vi "RSMA Receiver - 2 Channels - Kopie.vi"() -> ()   [LabVIEW 2022 SP3]
panel:
  out "W2":string
  out "W1":string
  out "Constellation Map":cluster{"Constellation":cdb[]}[](graph)
  in  "Tab Control":enum32{"USRP Parameters", "Rx Info", "BER"}(tab)
  in  "USRP ControledParameters":T1={"Active Antenna"="RX2", "Gain (dB)"=0.0, "Carrier Frequency"=2400000000.0, "IQ Rate"=2000000.0, "Active channels"="0,1"} {"IQ Rate" format="%#_6p"; "Carrier Frequency" format="%#_6p"; "Gain (dB)" format="%#_6f"}
  in  "Device selection":refnum<k15>="RIO0"
  in  "Trigger level":dbl=0.01 format="%f"
  out "SIG valid? - CH1":bool
  out "SIG valid? - CH0":bool
  out "Frequency offset - CH1":dbl
  out "Frequency offset - CH0":dbl
  out "Coerced Parameters":T2={"IQ Rate"=100000.0, "Carrier  Freq."=100000.0, "Gain"=0.0} {"Gain" format="%#_6f"; "Carrier  Freq." format="%#_6p"; "IQ Rate" format="%#_6p"}
  out "Error out":errorcluster
  in  "Record BER":bool
  out "No. Bits - CH0":dbl format="%#_6f"
  out "No. Bits - CH1":dbl
  in  "error in (no error)":errorcluster
  # "RSMA Receiver"
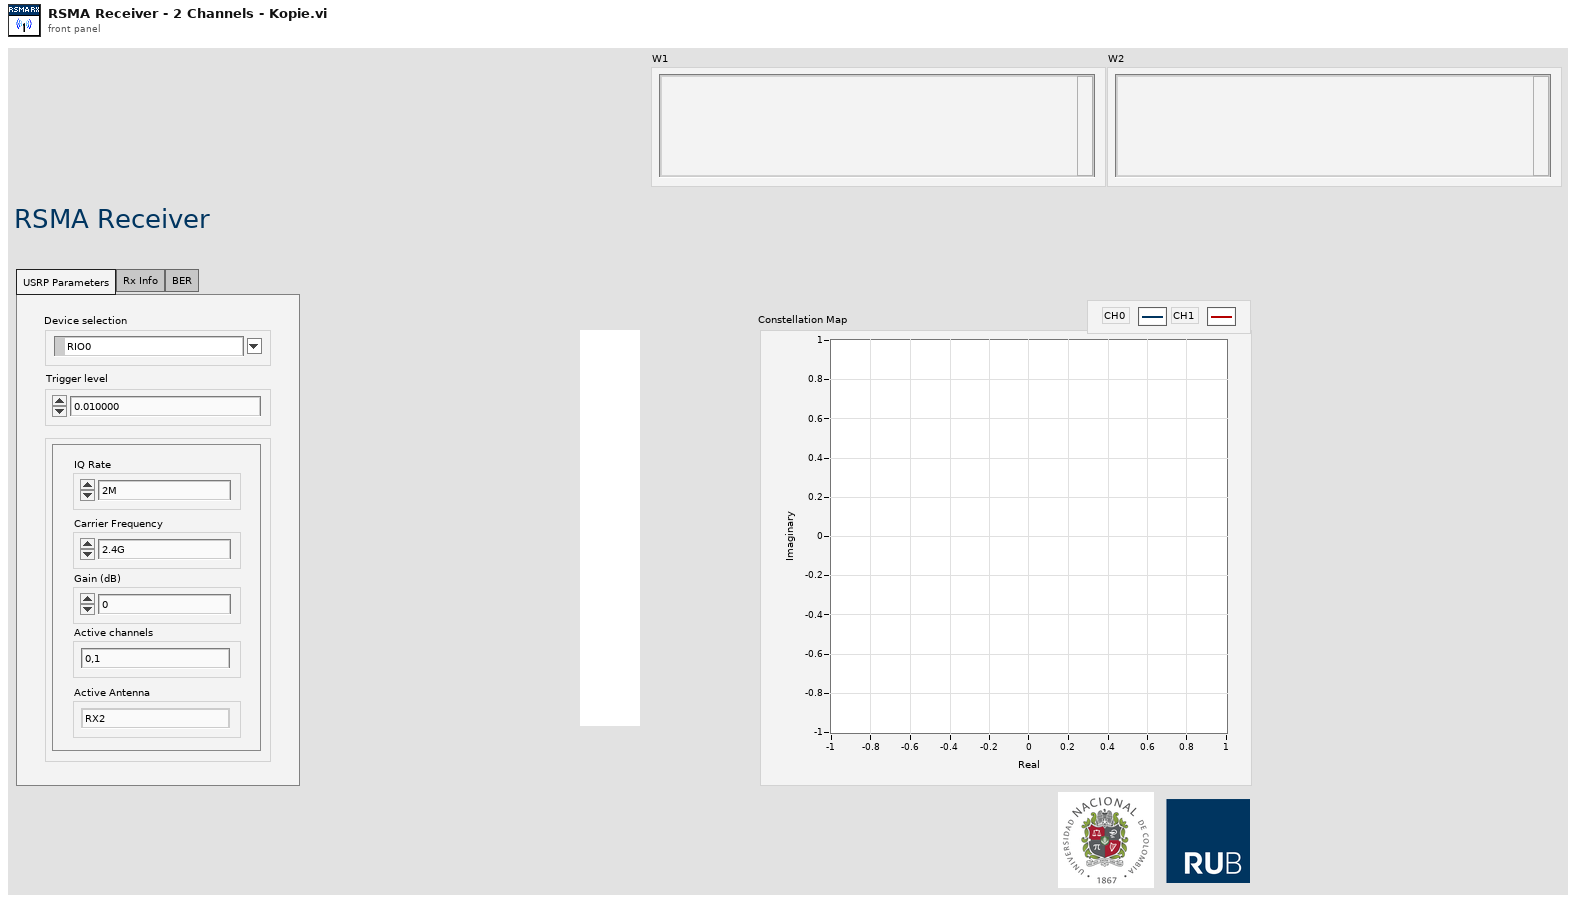
[diagram p1: front panel]
types:
  T1 = cluster{"Active Antenna":string, "Gain (dB)":dbl, "Carrier Frequency":dbl, "IQ Rate":dbl, "Active channels":string}
  T2 = cluster{"IQ Rate":dbl, "Carrier  Freq.":dbl, "Gain":dbl}
  T3 = cluster{"coerced IQ rate":dbl, "coerced carrier frequency":dbl, "coerced gain":dbl}
  T4 = cluster{"Modulation type":enum16{"QPSK(4QAM)", "64QAM", "16QAM", "BPSK"}, "BCC rate (k/n)":enum16{"1/2", "2/3", "3/4"}}
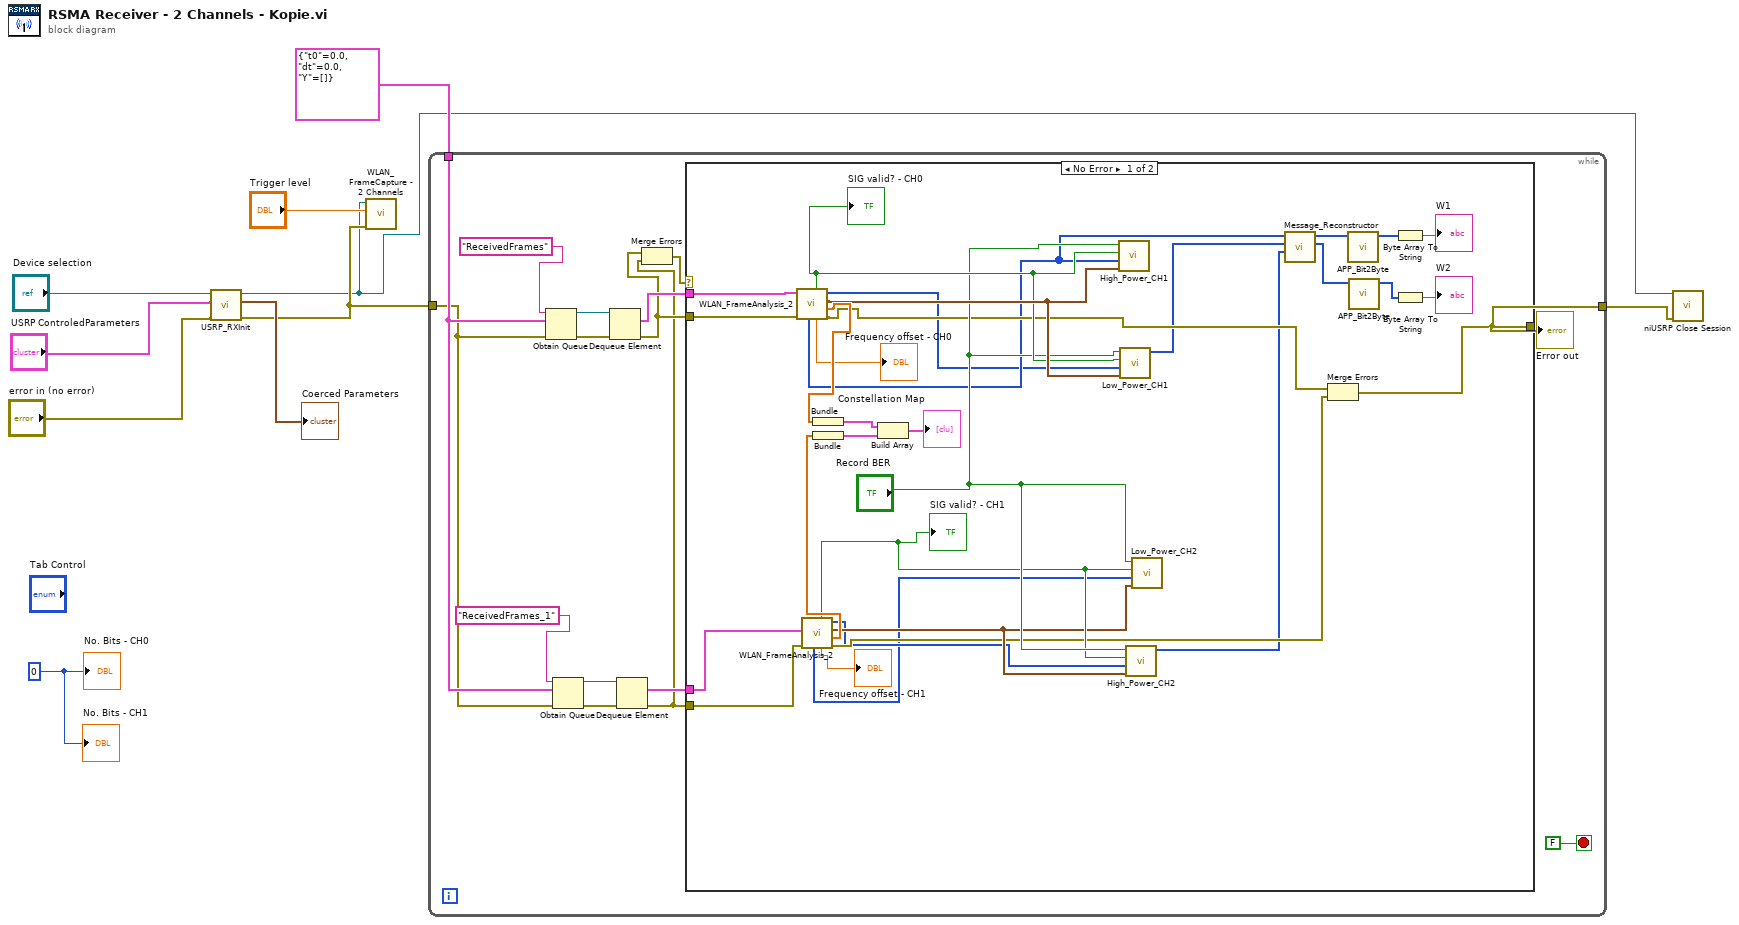
[diagram p0: block diagram]
diagram:
  w1 = 0
  n1 = call "USRP_RXInit.vi"("device names"="Device selection", "USRP ControledParameters"="USRP ControledParameters", "error in (no error)"="error in (no error)") -> ("session handle out"=w4:refnum<k15>, "USRP CoercedParamters"=→"Coerced Parameters":T3, "error out"=w8:errorcluster)  [unwired: 5 in]
  n2 = call "WLAN_FrameCapture - 2 Channels.vi"("error in (no error)"=w8, "Trigger level"="Trigger level", "session handle"=w4) -> ()  [unwired: 8 in]
  n3 = while {
    tunnel: w8 -> [w16]
    tunnel: cluster{"t0":dbl, "dt":dbl, "Y":cdb[]} {"t0"=0.0, "dt"=0.0, "Y"=[]} ("data") -> [w17]
    tunnel: [w21] -> w5
    stop <- FALSE stop-if-true
    n4 = Obtain Queue(name (unnamed)="ReceivedFrames", element data type=w17, error in (no error)=w16) -> (queue out=w25:refnum<queue>, error out=w23:errorcluster)  [unwired: 2 in, 1 out]
    n5 = Obtain Queue(name (unnamed)="ReceivedFrames_1", element data type=w17, error in (no error)=w16) -> (queue out=w20:refnum<queue>, error out=w19:errorcluster)  [unwired: 2 in, 1 out]
    n6 = Dequeue Element(queue=w25, error in (no error)=w23) -> (element=w24:cluster{"t0":dbl, "dt":dbl, "Y":cdb[]}, error out=w13:errorcluster)  [unwired: 1 in, 2 out]
    n7 = Dequeue Element(queue=w20, error in (no error)=w19) -> (element=w15:cluster{"t0":dbl, "dt":dbl, "Y":cdb[]}, error out=w12:errorcluster)  [unwired: 1 in, 2 out]
    n8 = Merge Errors(w13, w12) -> (w11:errorcluster)
    n9 = case shown="No Error" w11 {
      selector: w11 -> [_ w57]
      tunnel: w24 -> [w53 _]
      tunnel: [w38 w57] -> w21
      tunnel: w12 -> [w46 _]
      tunnel: w15 -> [w47 _]
      tunnel: w13 -> [w50 _]
      frame No Error {
        n10 = call "WLAN_FrameAnalysis_2.vi"("error in (no error)"=w50, "input cluster"=w53) -> ("error out"=w39:errorcluster, "Constellation"=w52:cdb[], "Modulation parameter"=w49:T4, "output bits"=w36:i8[], "Frequency offset"=→"Frequency offset - CH0":dbl, "SIG valid?"=w48:bool, "outputbitsHP"=w37:i8[])  [unwired: 3 in]
        "SIG valid? - CH0" <- w48
        n11 = call "WLAN_FrameAnalysis_2.vi"("error in (no error)"=w46, "input cluster"=w47) -> ("error out"=w40:errorcluster, "Constellation"=w44:cdb[], "Modulation parameter"=w41:T4, "output bits"=w28:i8[], "Frequency offset"=→"Frequency offset - CH1":dbl, "SIG valid?"=w42:bool, "outputbitsHP"=w27:i8[])  [unwired: 3 in]
        "SIG valid? - CH1" <- w42
        n12 = Bundle("Constellation"=w52) -> (w54:cluster{"Constellation":cdb[]})  [unwired: 1 in]
        n13 = Bundle("Constellation"=w44) -> (w55:cluster{"Constellation":cdb[]})  [unwired: 1 in]
        n14 = Build Array(w54, w55) -> (→"Constellation Map":cluster{"Constellation":cdb[]}[])
        n15 = call "High_Power_CH1.vi"("Modulation parameter"=w49, "output bits"=w37, "Boolean"=w48, "Record BER"="Record BER") -> ()  [unwired: 8 in]
        n16 = call "Low_Power_CH1.vi"("Modulation parameter"=w49, "output bits"=w36, "Boolean"=w48, "Record BER"="Record BER") -> ("subarray"=w26:i8[])  [unwired: 7 in]
        n17 = call "High_Power_CH2.vi"("Modulation parameter"=w41, "output bits"=w28, "Boolean"=w42, "Record BER"="Record BER") -> ("subarray2"=w35:i8[])  [unwired: 7 in]
        n18 = call "Low_Power_CH2.vi"("Modulation parameter"=w41, "output bits"=w27, "Boolean"=w42, "Record BER"="Record BER") -> ()  [unwired: 8 in]
        n19 = call "Message_Reconstructor.vi"("Wp2"=w35, "Wp1"=w26, "Wc"=w37) -> ("W2"=w30:u8[], "W1"=w31:u8[])  [unwired: 7 in]
        n20 = Merge Errors(w39, w40) -> (w38:errorcluster)
        n21 = call "APP_Bit2Byte.vi"("input bit stream"=w31) -> ("output byte stream"=w32:u8[])  [unwired: 10 in]
        n22 = call "APP_Bit2Byte.vi"("input bit stream"=w30) -> ("output byte stream"=w29:u8[])  [unwired: 10 in]
        n23 = Byte Array To String(unsigned byte array=w32) -> (string=→"W1":string)
        n24 = Byte Array To String(unsigned byte array=w29) -> (string=→"W2":string)
      }
      frame Error {
      }
    }
    "Error out" <- w21
  }
  n25 = call <instrlib>:"niUSRP Close Session.vi"("session handle"=w4, "error in (no error)"=w5) -> ()  [unwired: 13 in, 1 out]
  "No. Bits - CH0" <- w1
  "No. Bits - CH1" <- w1
